vi "Combine Status Monitor and Transient Capture (Single UUT).vi"() -> ()   [LabVIEW 2017]
uses:
  Status Monitor/Status Monitor (Single Unit).vi
  Status Monitor/Status Monitor Library.lvlib
panel:
  out "UUT Name":string
  in  "Soft Trigger":bool
  in  "Post-Trigger Samples":i32=100000
  in  "configuration file path":path
  in  "stop":bool
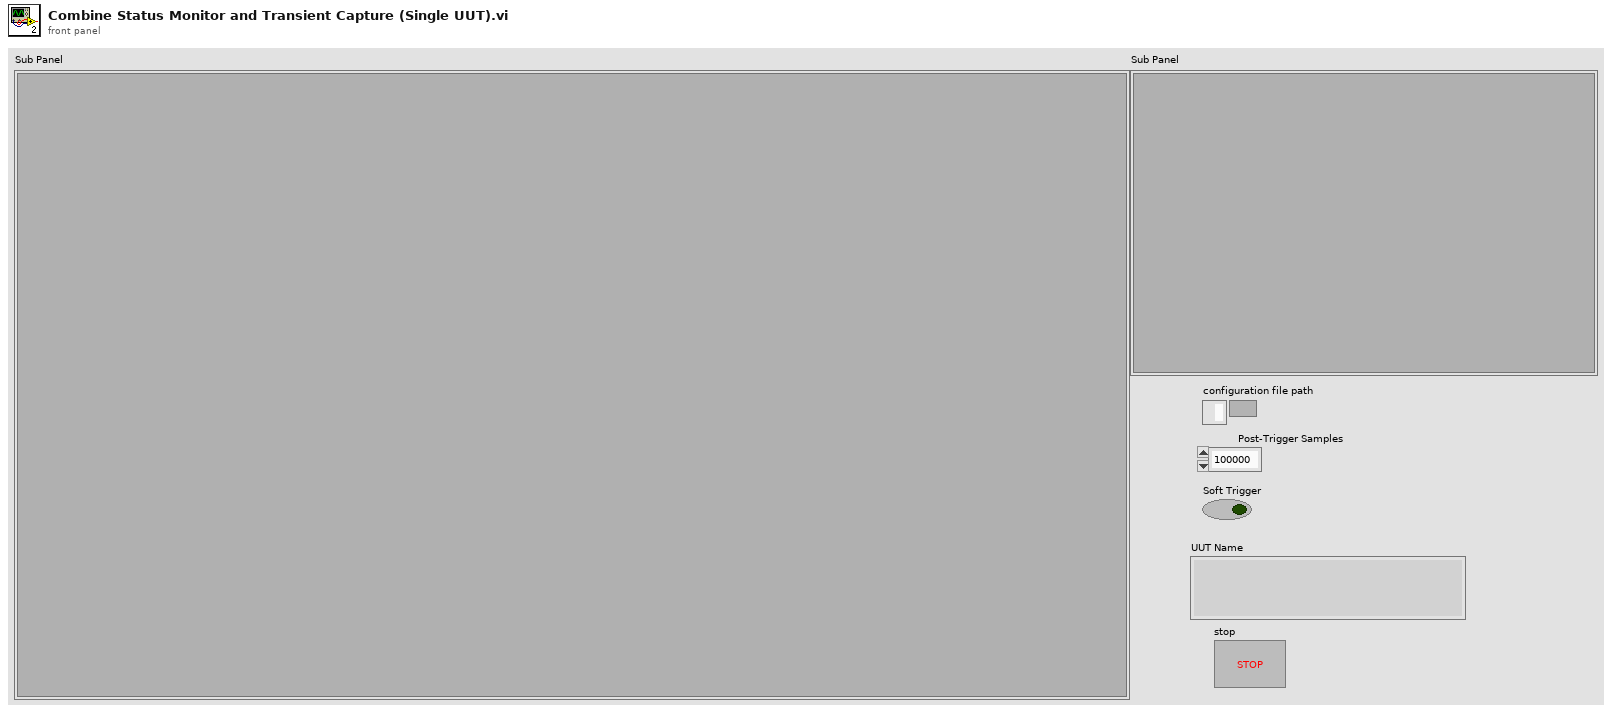
[diagram p1: front panel]
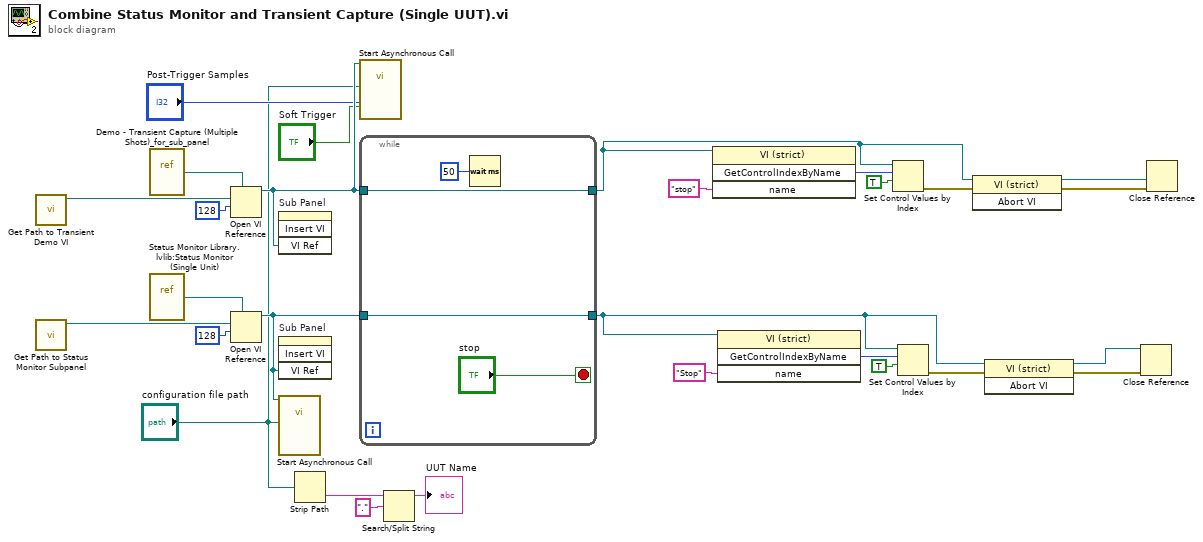
[diagram p0: block diagram]
diagram:
  n1 = call "Get Path to Transient Demo VI.vi"() -> ("Path to Transient Capture Subpanel"=w2:path)  [unwired: 11 in]
  n2 = call "Get Path to Status Monitor Subpanel.vi"() -> ("Path to Status Monitor Subpanel"=w1:path)  [unwired: 11 in]
  n3 = vi-ref "Demo - Transient Capture (Multiple Shots)_for_sub_panel.vi"() -> (w27:refnum<vi>)
  n4 = vi-ref "Status Monitor Library.lvlib:Status Monitor (Single Unit).vi"() -> (w24:refnum<vi>)
  n5 = Open VI Reference(type specifier VI Refnum (for type only)=w27, vi path=w2, options=128) -> (vi reference=w28:refnum<vi>)  [unwired: 3 in, 1 out]
  n6 = Open VI Reference(type specifier VI Refnum (for type only)=w24, vi path=w1, options=128) -> (vi reference=w23:refnum<vi>)  [unwired: 3 in, 1 out]
  n7 = invoke on="Sub Panel" class="SubPnl" method="Insert VI"("VI Ref"=w28) -> ()  [unwired: 3 in, 4 out]
  n8 = invoke on="Sub Panel" class="SubPnl" method="Insert VI"("VI Ref"=w23) -> ()  [unwired: 3 in, 4 out]
  n9 = call-by-ref "Start Asynchronous Call"(reference=w23, "configuration file path"="configuration file path") -> ()  [unwired: 12 in, 2 out]
  n10 = Strip Path(path="configuration file path") -> (name=w18:string)  [unwired: 1 out]
  n11 = call-by-ref "Start Asynchronous Call"(reference=w28, "Soft Trigger"="Soft Trigger", "Post-Trigger Samples"="Post-Trigger Samples", "configuration file path"="configuration file path") -> ()  [unwired: 10 in, 2 out]
  n12 = while {
    tunnel: w23 -> [w32]
    tunnel: w28 -> [w31]
    tunnel: [w32] -> w6
    tunnel: [w31] -> w9
    stop <- "stop" stop-if-true
    n13 = Wait (ms)(milliseconds to wait=u32 50) -> ()  [unwired: 1 out]
  }
  n14 = Search/Split String(string=w18, search string/char (-)=".") -> (substring before match=→"UUT Name":string)  [unwired: 1 in, 2 out]
  n15 = invoke class="VI (strict)" method="GetControlIndexByName"(reference=w9, "name"="stop") -> ("GetControlIndexByName"=w15:i32)  [unwired: 2 in, 3 out]
  n16 = invoke class="VI (strict)" method="GetControlIndexByName"(reference=w6, "name"="Stop") -> ("GetControlIndexByName"=w12:i32)  [unwired: 2 in, 3 out]
  n17 = Set Control Values by Index(0:w9, 1:w15, 2:TRUE) -> (11:w7:errorcluster)  [unwired: 1 in]
  n18 = Set Control Values by Index(0:w6, 1:w12, 2:TRUE) -> (11:w5:errorcluster)  [unwired: 1 in]
  n19 = invoke class="VI (strict)" method="Abort VI"(reference=w9, error in=w7) -> (reference out=w10:refnum<vi>, error out=w8:errorcluster)  [unwired: 1 in, 1 out]
  n20 = invoke class="VI (strict)" method="Abort VI"(reference=w6, error in=w5) -> (reference out=w3:refnum<vi>, error out=w4:errorcluster)  [unwired: 1 in, 1 out]
  n21 = Close Reference(reference=w3, error in (no error)=w4) -> ()  [unwired: 1 out]
  n22 = Close Reference(reference=w10, error in (no error)=w8) -> ()  [unwired: 1 out]
